vi "10pt Mov Avg.vi"(10 "Value in":dbl) -> (2 "Value out":dbl)   [LabVIEW 2014]
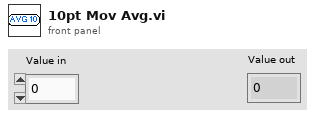
[diagram p1: front panel]
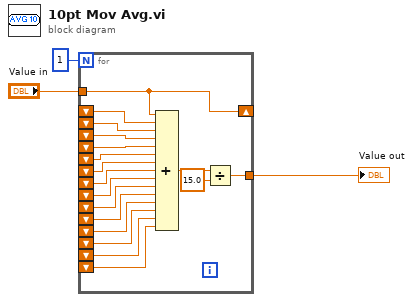
[diagram p0: block diagram]
diagram:
  n1 = for {
    N: 1 -> [_]
    tunnel: "Value in" -> [w21]
    shift-right: [w21] -> _
    shift-left: _ -> [w20]
    shift-left: _ -> [w19]
    shift-left: _ -> [w18]
    shift-left: _ -> [w17]
    tunnel: [w14] -> w1
    shift-left: _ -> [w13]
    shift-left: _ -> [w12]
    shift-left: _ -> [w11]
    shift-left: _ -> [w10]
    shift-left: _ -> [w9]
    shift-left: _ -> [w8]
    shift-left: _ -> [w7]
    shift-left: _ -> [w6]
    shift-left: _ -> [w5]
    shift-left: _ -> [w4]
    n2 = Compound Arithmetic op=ADD(w21, w20, w19, w18, w17, w13, w12, w11, w10, w9, w8, w7, w6, w5, w4) -> (w16:dbl)
    n3 = Divide(x=w16, y=15.0) -> (x/y=w14:dbl)
  }
  "Value out" <- w1
